vi "Gen Mult Voltage Updates.vi"() -> ()   [LabVIEW 2021]
doc: "I. Description:\nThis example demonstrates how to output a single Voltage Update (Sample) to an Analog Output Channel.\n\nII. Instructions for Running:\n1. Select the Physical Channel to correspond to where your signal is output on the DAQ device.\n2. Enter the Minimum and Maximum Voltage Ranges\nNote: Use the Acq One Sample example to verify you are generating the correct output on the DAQ device\n\nIII. Block Diagram Steps:\n1. Create an Analog Output Voltage Channel\n2. Use the Write VI to Output 1 Sample to 1 Channel on the Data\nAcquisition Card. \n3. Call the Clear Task VI to clear the Task.\n4. Use the popup dialog box to display an error if any. \n\nIV. I/O Connections Overview:\nMake sure your signal output terminal matches the Physical Channel I/O Control. For further connection information, refer to your hardware reference manual."
uses:
  <vilib>/userdefined/High Color/nirio_resource_hc.ctl
  <vilib>/FPGAPlugInAG/PCIe-7857/niLvFpga_Open_PCIe-7857.vi
  <vilib>/rvi/interface/common/dynamic/niFpgaDynamicAddResources.vi
  <vilib>/Utility/error.llb/Error Cluster From Error Code.vi
  <vilib>/rvi/errors/niLvFpgaAdjustHostInterfaceError.vi
  <vilib>/FPGAPlugInAG/Dynamic/niLvFpga_Close_Dynamic.vi
  <vilib>/rvi/interface/nirviOpenFPGA/nirviOpenFPGA.xnode
  FPGA Bitfiles/lvfpga_FPGATarget_AO_PspK-PiI6Y0.lvbitx
  AO.vi
  <vilib>/rvi/interface/nirviReadWriteControl/nirviReadWriteControl.xnode
  <vilib>/rvi/interface/nirviCloseFPGA/nirviCloseFPGA.xnode
  NiFpgaLv.dll
  <vilib>/rvi/interface/Simulation/niFpgaSimulationCallBeginRW.vi
panel:
  in  "RIO Resource Name":T1="RIO0" caption="RIO Device"
  in  "AO Channels":dbl[](array[slide]) scale=-10.0..9.995 scale format="%.1f"
  in  "stop":bool
  # "Channel Parameters"
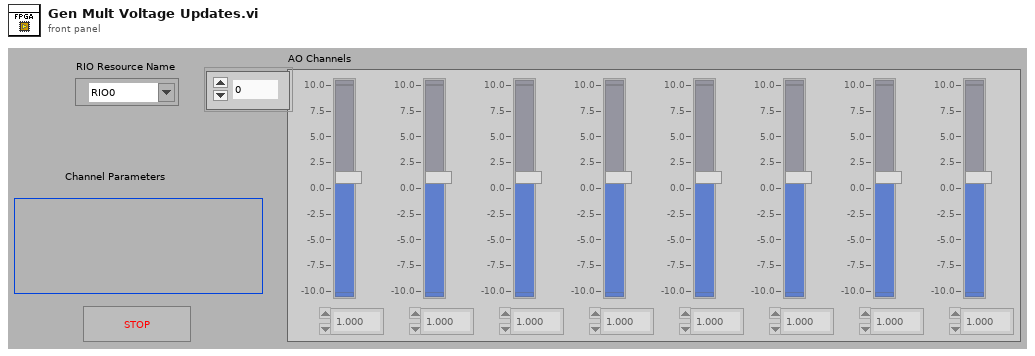
[diagram p1: front panel]
types:
  T1 = typedef "nirio_resource_hc.ctl" = tag
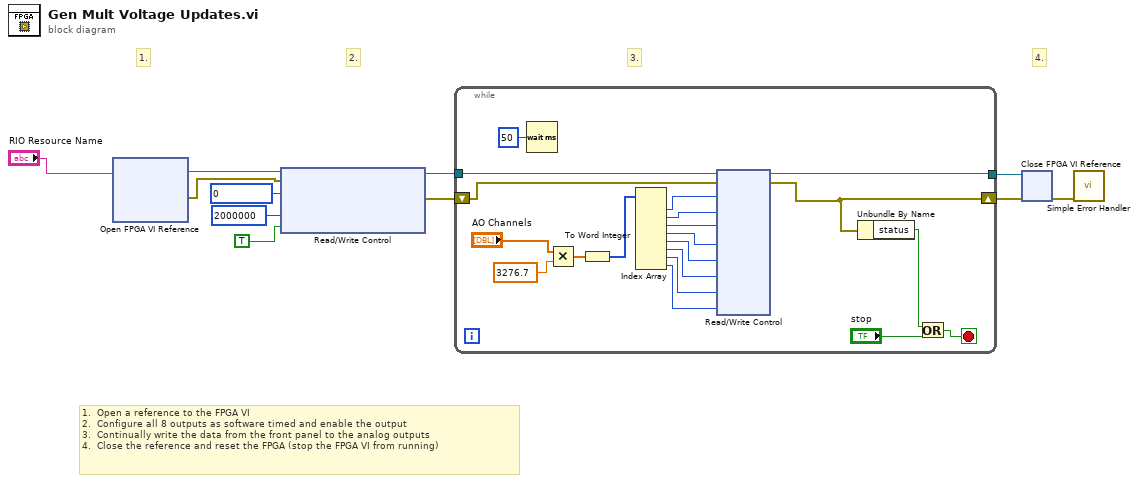
[diagram p0: block diagram]
diagram:
  # "1.  Open a reference to the FPGA VI\n2.  Configure all 8 outputs as software timed and enable the output\n3.  Continually write the data from the front panel to the analog outputs\n4.  Close the reference and reset the FPGA (stop the FPGA VI from running)"
  # "4."
  # "3."
  # "2."
  # "1."
  n1 = xnode "Open FPGA VI Reference"("resource name"="RIO Resource Name") -> ("FPGA VI Reference Out"=w5:refnum<k20>, "error out"=w6:errorcluster)  [unwired: 1 in]
  n2 = xnode "Read/Write Control"("FPGA VI Reference In"=w5, "error in"=w6, "AO Buffer Enable"=u8 0, "AO Loop Timer(Ticks)"=u32 2000000, "AO Enable"=TRUE) -> ("FPGA VI Reference Out"=w8:refnum<k20>, "error out"=w7:errorcluster)
  n3 = while {
    tunnel: w8 -> [w31]
    shift-right: [w21] -> w10
    shift-left: w7 -> [w30]
    tunnel: [w22] -> w11
    stop <- w23 stop-if-true
    n4 = Wait (ms)(milliseconds to wait=u32 50) -> ()  [unwired: 1 out]
    n5 = Multiply(x="AO Channels", y=3276.7) -> (x*y=w28:dbl[])
    n6 = To Word Integer(number=w28) -> (16bit integer=w27:i16[])
    n7 = Index Array(array=w27) -> (element #1=w19:i16, element #2=w18:i16, element #3=w17:i16, element #4=w16:i16, element #5=w15:i16, element #6=w14:i16, element #7=w13:i16, element #8=w12:i16)  [unwired: 8 in]
    n8 = xnode "Read/Write Control"("FPGA VI Reference In"=w31, "error in"=w30, "AO 0"=w19, "AO 1"=w18, "AO 2"=w17, "AO 3"=w16, "AO 4"=w15, "AO 5"=w14, "AO 6"=w13, "AO 7"=w12) -> ("FPGA VI Reference Out"=w22:refnum<k20>, "error out"=w21:errorcluster)
    n9 = Unbundle By Name(w21) -> ("status"=w24:bool)
    n10 = Or(x=w24, y="stop") -> (x .or. y?=w23:bool)
  }
  n11 = xnode "Close FPGA VI Reference"("FPGA VI Reference In"=w11, "error in"=w10) -> ("error out"=w9:errorcluster)
  n12 = call <vilib>:"Simple Error Handler.vi"("error in (no error)"=w9) -> ()  [unwired: 4 in, 5 out]
